vi "2D Quadrature (Formula).vi"(8 "tolerance":dbl=1e-05, 9 "Lower Limits":T1, 10 "Upper Limits":T2={"x upper limit"=1.0, "y upper limit"=1.0}, 11 "integrand":string) -> (0 "error":i32, 3 "result":dbl)   [LabVIEW 2017, in "NI_AALPro.lvlib"]
doc: "Performs numerical integration using adaptive quadrature approach. You must manually select the polymorphic instance to use."
uses:
  <vilib>/Analysis/NI_AALPro.lvlib
panel:
  # "Use x,y as the independent variable in integrand.\nExample:\nintegrand:  sin(x+y)\nx upper = 1, x lower = 0, \ny upper = 1, y lower = 0,\nresult = 0.773645"
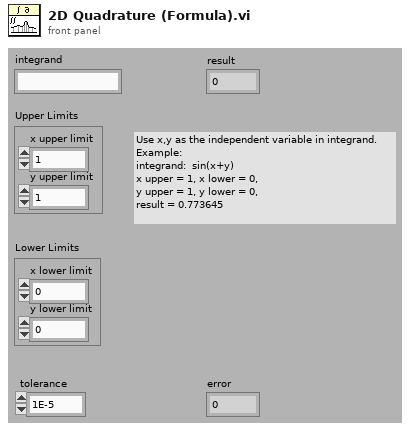
[diagram p1: front panel]
types:
  T1 = cluster{"x lower limit":dbl, "y lower limit":dbl}
  T2 = cluster{"x upper limit":dbl, "y upper limit":dbl}
  T3 = cluster{"x lower limit":dbl, "x upper limit":dbl}
  T4 = cluster{"y lower limit":dbl, "y upper limit":dbl}
  T5 = cluster{cluster{"x lower limit":dbl, "x upper limit":dbl}, cluster{"y lower limit":dbl, "y upper limit":dbl}}
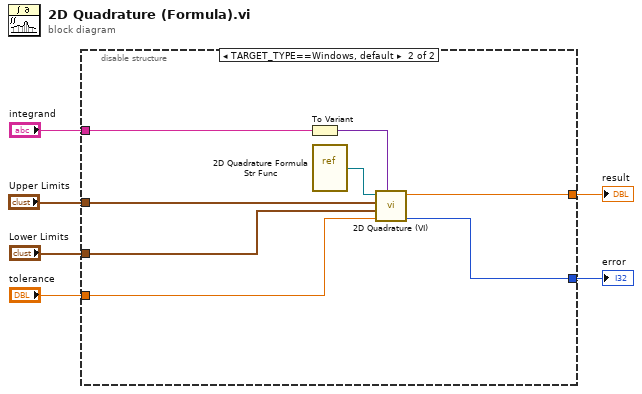
[diagram p0: block diagram]
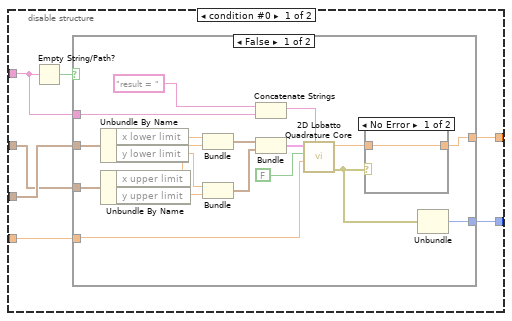
[diagram p2: hidden frame]
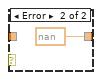
[diagram p3: hidden frame]
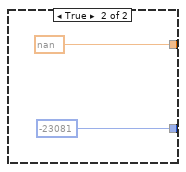
[diagram p4: hidden frame]
diagram:
  n1 = disable-structure shown="TARGET_TYPE==Windows, default" {
    disable-tunnel: [w12 w39] -> w1
    disable-tunnel: "integrand" -> [w11 w37]
    disable-tunnel: "Upper Limits" -> [w7 w43]
    disable-tunnel: "Lower Limits" -> [w8 w42]
    disable-tunnel: "tolerance" -> [w10 w41]
    disable-tunnel: [w9 w40] -> w2
    frame condition #0 {
      n2 = Empty String/Path?(string/path=w11) -> (empty?=w13:bool)
      n3 = case shown="False" w13 {
        tunnel: [w30 nan] -> w9
        tunnel: [w29 -23081] -> w12
        tunnel: w11 -> [w28 _]
        tunnel: w8 -> [w20 _]
        tunnel: w7 -> [w19 _]
        tunnel: w10 -> [w14 _]
        frame False {
          n4 = Unbundle By Name(w20) -> ("x lower limit"=w26:dbl, "y lower limit"=w22:dbl)
          n5 = Unbundle By Name(w19) -> ("x upper limit"=w25:dbl, "y upper limit"=w23:dbl)
          n6 = Bundle("x lower limit"=w26, "x upper limit"=w25) -> (w24:T3)  [unwired: 1 in]
          n7 = Bundle("y lower limit"=w22, "y upper limit"=w23) -> (w21:T4)  [unwired: 1 in]
          n8 = Concatenate Strings("result = ", w28) -> (w17:string)
          n9 = Bundle(w24, w21) -> (w16:T5)  [unwired: 1 in]
          n10 = call <vilib>:"2D Lobatto Quadrature Core.vi"("formula"=w17, "tolerance"=w14, "Formula/VI ref"=FALSE, "limits"=w16) -> ("error out"=w27:errorcluster, "result"=w31:dbl)  [unwired: 6 in]
          n11 = case shown="No Error" w27 {
            tunnel: w31 -> [w32 _]
            tunnel: [w32 nan] -> w30
            frame No Error {
            }
            frame Error {
            }
          }
          n12 = Unbundle(w27) -> ("code"=w29:i32)  [unwired: 2 out]
        }
        frame True {
        }
      }
    }
    frame condition #1 (active) {
      n13 = To Variant(anything=w37) -> (Variant=w38:variant)
      n14 = vi-ref <vilib>:"2D Quadrature Formula Str Func.vi"() -> (w36:refnum<vi>)
      n15 = call <vilib>:"2D Quadrature (VI).vi"("data"=w38, "tolerance"=w41, "Lower Limits"=w42, "Upper Limits"=w43, "integrand"=w36) -> ("error"=w39:i32, "result"=w40:dbl)  [unwired: 5 out]
    }
  }
  "error" <- w1
  "result" <- w2
